vi "GT Arc ZXR Override2WN.vi"(0 "cardNum":i16, 1 "radius":dbl, 2 "synVel":dbl, 3 "velEnd":dbl, 5 "crd":i16, 7 "z":i32, 9 "x":i32, 10 "fifo":i16, 11 "error in (no error)":errorcluster caption="错误输入（无错误）", 12 "circleDir":i16, 13 "synAcc":dbl, 14 "segNum":i32) -> (4 "function return":i16, 15 "error out":errorcluster caption="错误输出")   [LabVIEW 2020, in "gts.lvlib"]
doc: "GT_API GT_ArcZXROverride2WN(short cardNum,short crd,long z,long x,double radius,short circleDir,double synVel,double synAcc,double velEnd=0,long segNum=0,short fifo=0);"
uses:
  gts.lvlib
  dll/32bit/multi_card/gts.dll
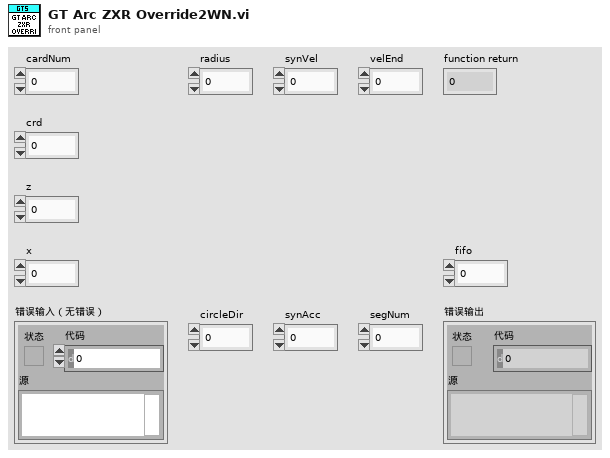
[diagram p1: front panel]
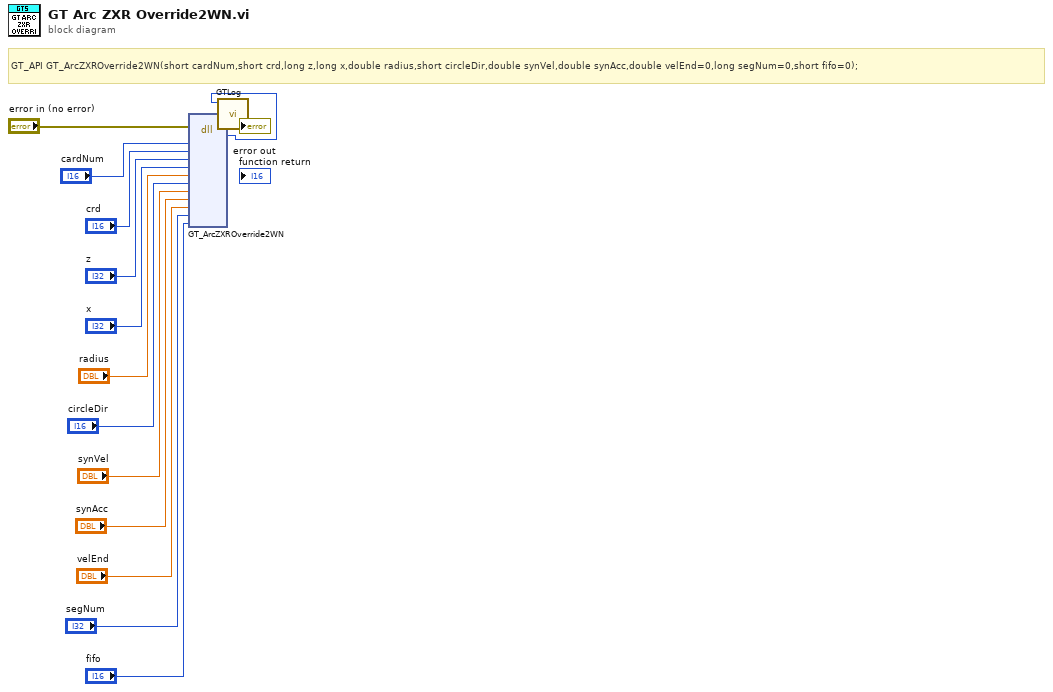
[diagram p0: block diagram]
diagram:
  # "GT_API GT_ArcZXROverride2WN(short cardNum,short crd,long z,long x,double radius,short circleDir,double synVel,double synAcc,double velEnd=0,long segNum=0,short fifo=0);"
  n1 = dll-call lib="C:/1228/dll/32bit/multi_card/gts.dll" fn="GT_ArcZXROverride2WN"(error in="error in (no error)", "cardNum"="cardNum", "crd"="crd", "z"="z", "x"="x", "radius"="radius", "circleDir"="circleDir", "synVel"="synVel", "synAcc"="synAcc", "velEnd"="velEnd", "segNum"="segNum", "fifo"="fifo") -> (error out=w3:errorcluster, w1:i16)  [unwired: 13 in, 1 out]
  n2 = call "GTLog.vi"("error in (no error)"=w3, "Numeric"=w1) -> ("error out"=→"error out":errorcluster)  [unwired: 9 in]
